vi "Extract Band Diagram from Atoms and DOS.vi"(6 "Low Density Cutoff":dbl, 8 "Style":enum16{"Linear Step", "Linear Pts", "Log Pts"}(ring), 9 "Step or #pts":dbl, 10 "DOS Parsed":T2(array[cluster]), 11 "Structure":T1) -> (2 "All Energy vs DOS by Z":cluster{"DOS":dbl[], dbl[]}[](graph), 3 "Band Edge Diagram":cluster{"Array":dbl[], dbl[]}[](graph))   [LabVIEW 2010]
panel:
  # "Energy,Total,"
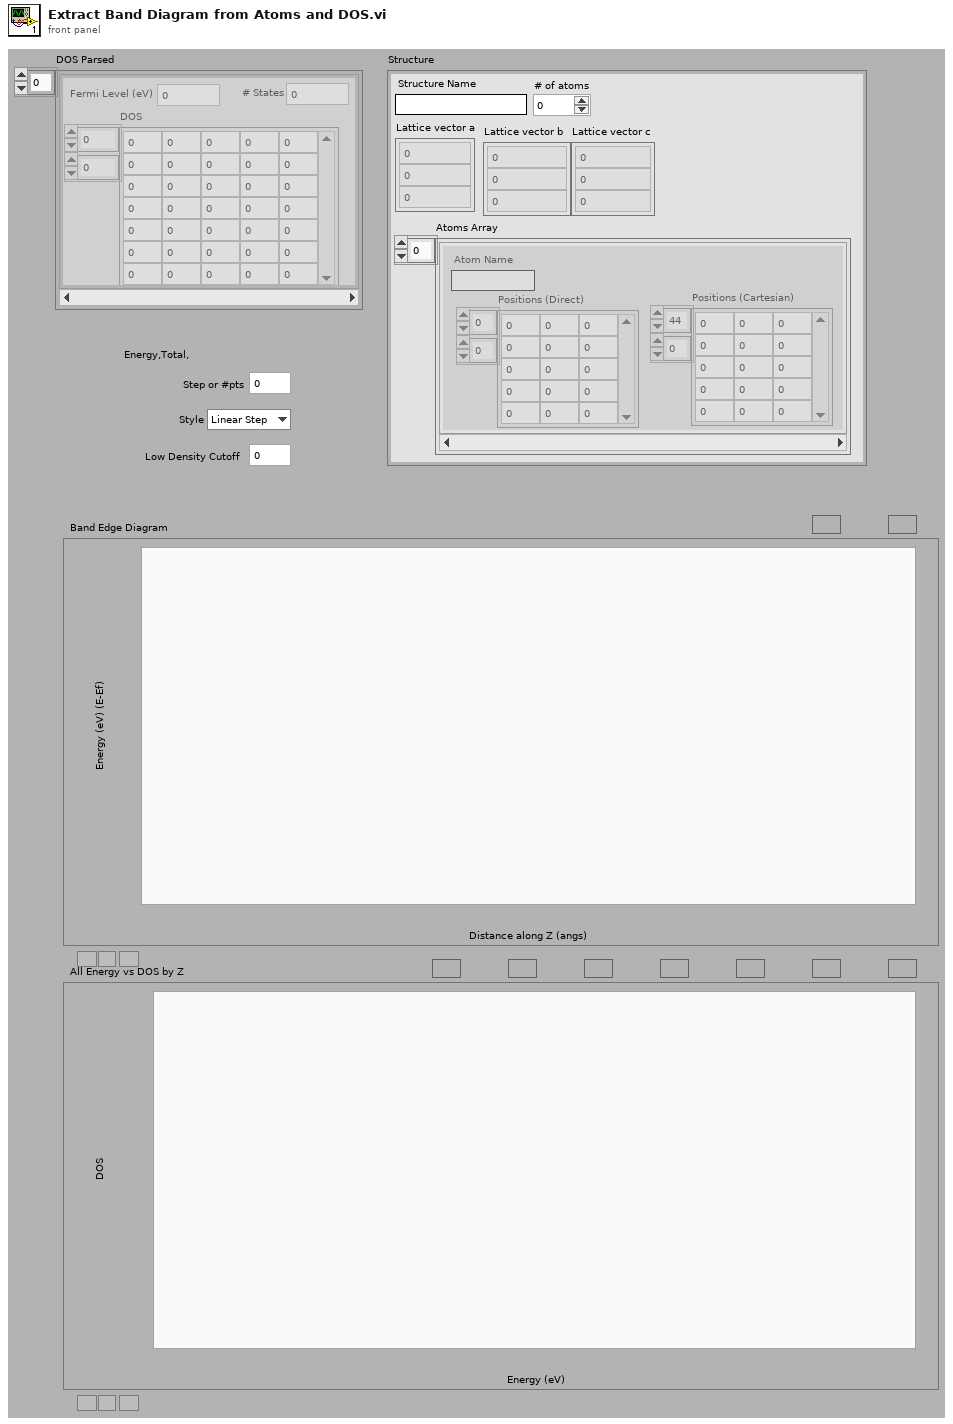
[diagram p1: front panel]
types:
  T1 = cluster{"Structure Name":string, "Lattice vector a":dbl[], "Lattice vector b":dbl[], "Lattice vector c":dbl[], "Atoms Array":cluster{"Atom Name":string, "Positions (Direct)":dbl[][], "Positions (Cartesian)":dbl[][]}[], "# of atoms":i32}
  T2 = cluster{"Fermi Level (eV)":dbl, "# States":dbl, "DOS":dbl[][]}[]
  T3 = cluster{"Fermi Level (eV)":dbl, "# States":dbl, "DOS":dbl[][]}
  T4 = cluster{"Atom Name":string, "Positions (Direct)":dbl[][], "Positions (Cartesian)":dbl[][]}[]
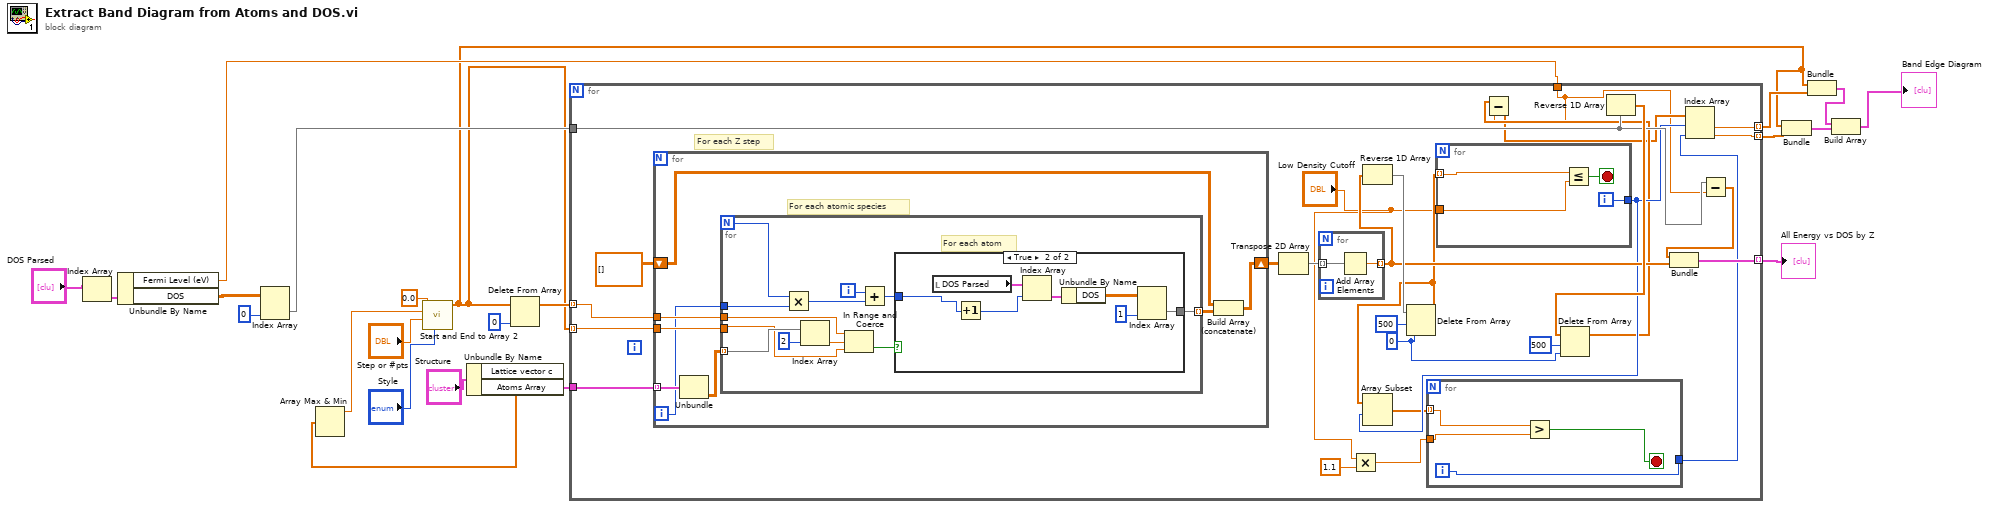
[diagram p0: block diagram]
diagram:
  n1 = Index Array(array="DOS Parsed") -> (element=w19:T3)  [unwired: 1 in]
  n2 = Unbundle By Name(w19) -> ("Fermi Level (eV)"=w7:dbl, "DOS"=w18:dbl[][])
  n3 = Index Array(array=w18, index (col)=0 ("disabled index (col)")) -> (element=w12:dbl[])  [unwired: 1 in]
  n4 = Unbundle By Name("Structure") -> ("Lattice vector c"=w10:dbl[], "Atoms Array"=w21:T4)
  n5 = Array Max & Min(array=w10) -> (max value=w9:dbl)  [unwired: 3 out]
  n6 = call "Start and End to Array 2.vi"("Sweep Style"="Style", "Step or # Pts"="Step or #pts", "End"=w9, "Start"=0.0) -> ("Array"=w3:dbl[])  [unwired: 7 in]
  n7 = Delete From Array(array=w3, index=0) -> (array with subset deleted=w13:dbl[])  [unwired: 1 in, 1 out]
  n8 = for {
    tunnel: w21 -> [w49]
    tunnel: w3 -> [w48] mode=indexing
    tunnel: w13 -> [w47] mode=indexing
    tunnel: [w30] -> w6 mode=indexing
    tunnel: w12 -> [w36]
    tunnel: [w44] -> w11 mode=indexing
    tunnel: w7 -> [w27]
    tunnel: [w26] -> w4 mode=indexing
    w38 = 0 ("index")
    # "For each Z step"
    n9 = for {
      tunnel: w49 -> [w67] mode=indexing
      tunnel: w48 -> [w65]
      tunnel: w47 -> [w64]
      shift-right: [w62] -> w43
      shift-left: dbl[][] [] -> [w61]
      i -> [w60]
      # "For each atomic species"
      n10 = Unbundle(w67) -> ("Positions (Cartesian)"=w66:dbl[][])  [unwired: 2 out]
      n11 = for {
        N -> [w75]
        tunnel: w66 -> [w79] mode=indexing
        tunnel: w60 -> [w74]
        tunnel: w65 -> [w70]
        tunnel: w64 -> [w71]
        tunnel: [w69] -> w63 mode=indexing
        i -> [w76]
        # "For each atom"
        n12 = Multiply(x=w75, y=w74) -> (x*y=w73:i32)
        n13 = Index Array(array=w79, index=2) -> (element=w77:dbl)
        n14 = In Range and Coerce(upper limit=w71, x=w77, lower limit=w70) -> (In Range?=w68:bool)  [unwired: 1 out]
        n15 = Add(x=w76, y=w73) -> (x+y=w72:i32)
        n16 = case shown="True" w68 {
          tunnel: w72 -> [_ w81]
          tunnel: [_ w82] -> w69
          frame False {
          }
          frame True {
            n17 = local read "DOS Parsed"() -> (w85:T2)
            n18 = Increment(x=w81) -> (x+1=w80:i32)
            n19 = Index Array(array=w85, index=w80) -> (element=w86:T3)
            n20 = Unbundle By Name(w86) -> ("DOS"=w84:dbl[][])
            n21 = Index Array(array=w84, index (col)=1 ("disabled index (col)")) -> (element=w82:dbl[])  [unwired: 1 in]
          }
        }
      }
      n22 = Build Array (concatenate)(w61, w63) -> (w62:dbl[][])
    }
    n23 = Transpose 2D Array(2D array=w43) -> (transposed array=w46:dbl[][])
    n24 = for {
      tunnel: w46 -> [w59] mode=indexing
      tunnel: [w58] -> w37 mode=indexing
      n25 = Add Array Elements(numeric array=w59) -> (sum=w58:dbl)
    }
    n26 = Multiply(x="Low Density Cutoff", y=1.1) -> (x*y=w23:dbl)
    n27 = Reverse 1D Array(array=w37) -> (reversed array=w42:dbl[])
    n28 = Delete From Array(array=w42, length=500, index=w38) -> (array with subset deleted=w34:dbl[])  [unwired: 1 out]
    n29 = for {
      tunnel: w34 -> [w57] mode=indexing
      tunnel: [w55] -> w33
      tunnel: "Low Density Cutoff" -> [w54]
      i -> [w55]
      stop <- w56 stop-if-true
      n30 = Less Or Equal?(x=w57, y=w54) -> (x <= y?=w56:bool)
    }
    n31 = Array Subset(array=w34, index=w33) -> (w32:dbl[])  [unwired: 1 in]
    n32 = for {
      tunnel: w32 -> [w53] mode=indexing
      tunnel: w23 -> [w52]
      tunnel: [w50] -> w31
      i -> [w50]
      stop <- w51 stop-if-true
      n33 = Greater?(x=w53, y=w52) -> (0:w51:bool)
    }
    n34 = Reverse 1D Array(array=w36) -> (reversed array=w39:dbl[])
    n35 = Delete From Array(array=w39, length=500, index=w38) -> (array with subset deleted=w29:dbl[])  [unwired: 1 out]
    n36 = Subtract(x=w29, y=w27) -> (x-y=w28:dbl[])
    n37 = Index Array(array=w28, index #1=w33, index #2=w31) -> (element #1=w30:dbl, element #2=w26:dbl)
    n38 = Subtract(x=w36, y=w27) -> (x-y=w35:dbl[])
    n39 = Bundle(w35, w37) -> (w44:cluster{dbl[], dbl[]})  [unwired: 1 in]
  }
  "All Energy vs DOS by Z" <- w11
  n40 = Bundle("Array"=w3, w4) -> (w2:cluster{"Array":dbl[], dbl[]})  [unwired: 1 in]
  n41 = Bundle("Array"=w3, w6) -> (w5:cluster{"Array":dbl[], dbl[]})  [unwired: 1 in]
  n42 = Build Array(w5, w2) -> (→"Band Edge Diagram":cluster{"Array":dbl[], dbl[]}[])
